vi "ReadTangoTestLongAttributes.vi"() -> ()   [LabVIEW 2009]
uses:
  tango_lv8/tango_vi.llb/ReadLongScalarAttribute.vi
  tango_lv8/tango_vi.llb/ReadLongSpectrumAttribute.vi
  tango_lv8/tango_vi.llb/ReadLongImageAttribute.vi
panel:
  out "?":bool
  out "scalar attr. read (RO)":i32
  out "Read/s":dbl
  in  "?":bool=TRUE
  out "Read/s":dbl
  out "Read/s":dbl
  in  "?":bool=TRUE
  in  "?":bool=TRUE
  out "Read/s":dbl
  in  "?":bool=TRUE
  out "error stack":string[](array[string])
  out "error stack":string[](array[string])
  out "error stack":string[](array[string])
  out "scalar attr. value":i32(graph)
  out "scalar attr. write value":i32
  out "scalar attr. read value":i32
  out "?":bool
  in  "attr_name":string="long_scalar"
  out "?":bool
  in  "attr_name":string="long_spectrum_ro"
  out "?":bool
  out "image attr. value":i32[][](graph)
  out "spectrum attr. value":i32[](graph)
  in  "attr_name":string="long_image_ro"
  in  "dev_name":string="tango/tangotest/1"
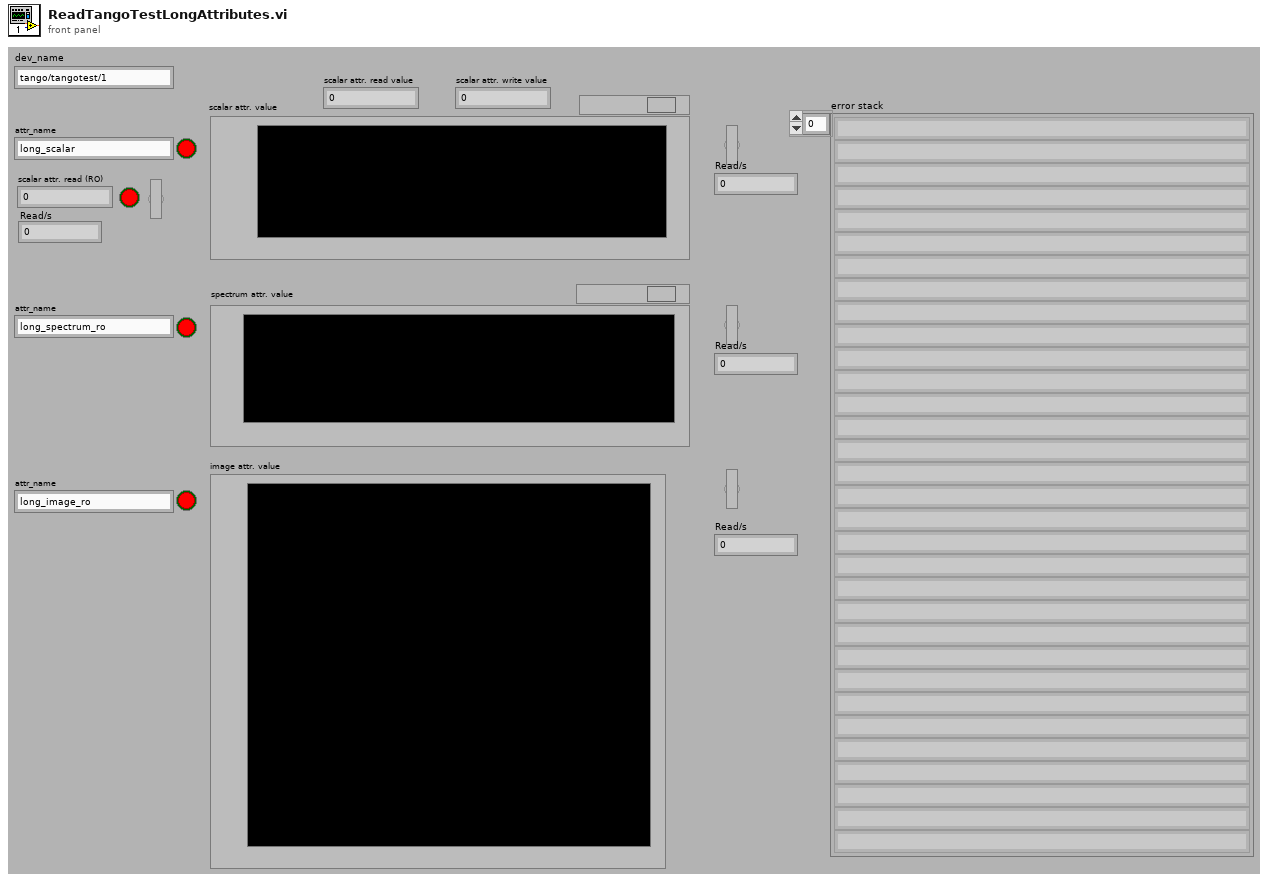
[diagram p1: front panel]
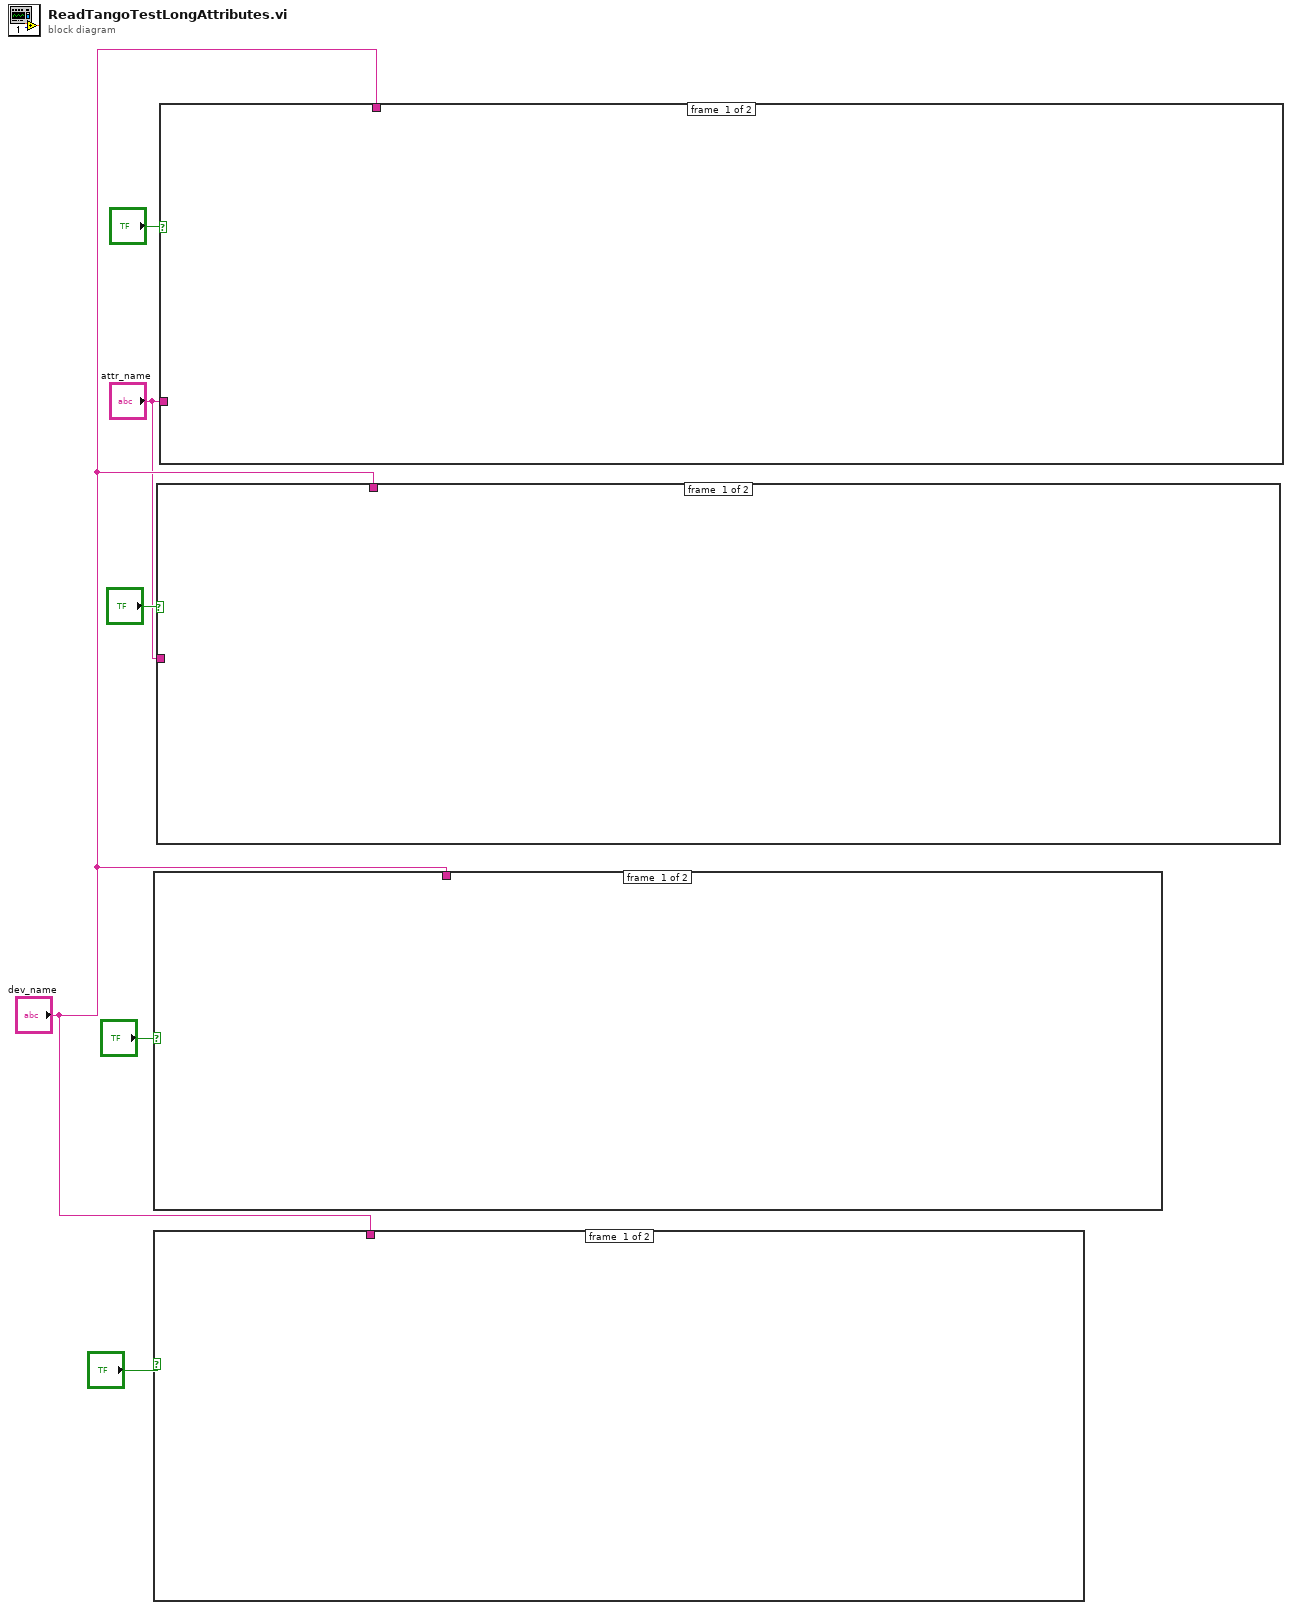
[diagram p0: block diagram]
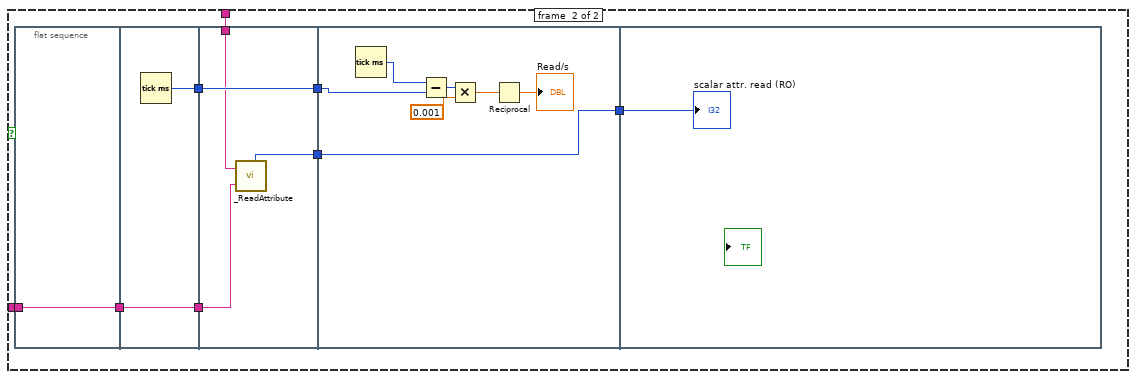
[diagram p2: hidden frame]
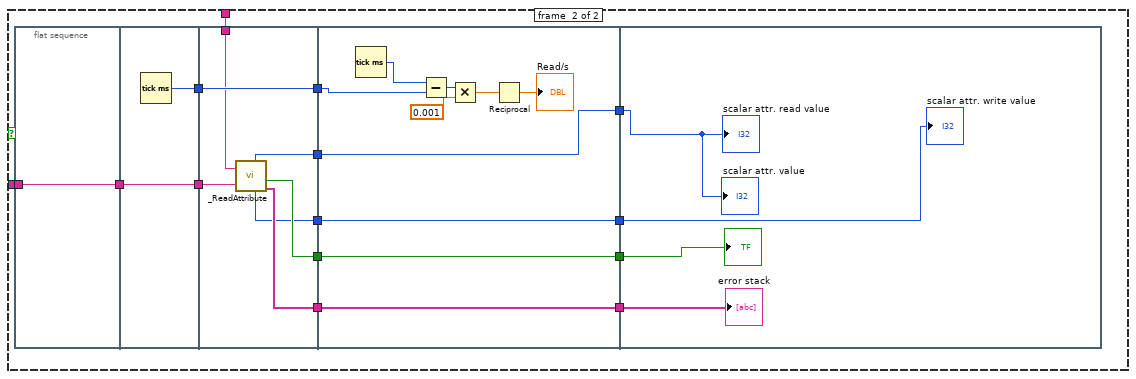
[diagram p3: hidden frame]
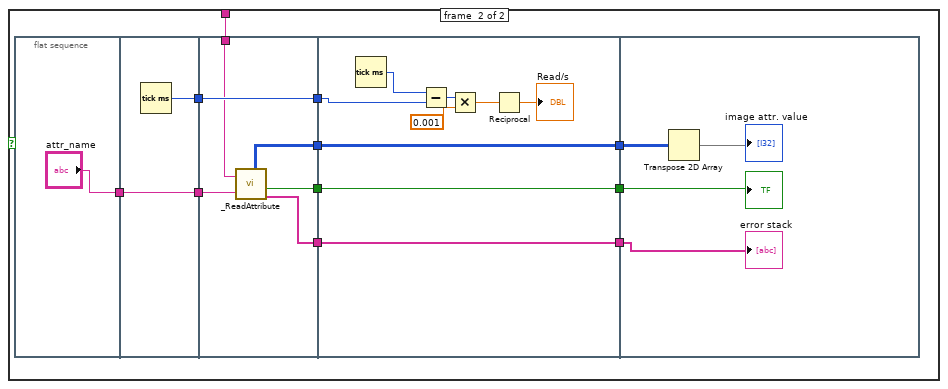
[diagram p4: hidden frame]
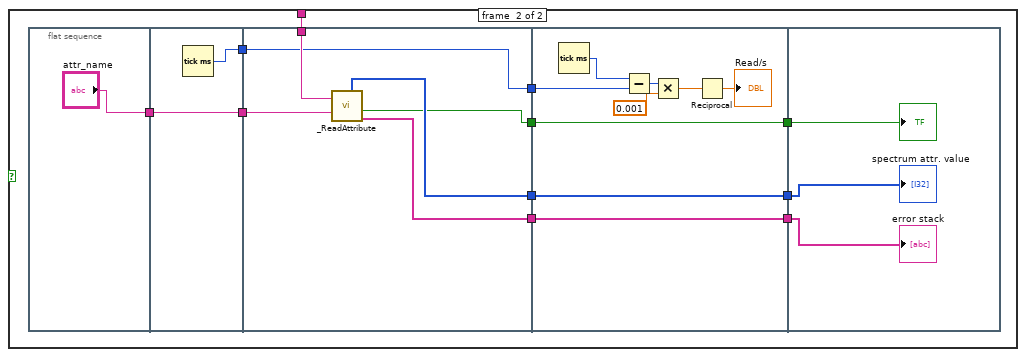
[diagram p5: hidden frame]
diagram:
  n1 = case shown="True" "?" {
    tunnel: "dev_name" -> [_ w9]
    frame #0 {
    }
    frame #1 {
      n2 = flat-sequence {
        tunnel: ["attr_name"] -> w17
        tunnel: [w20] -> w16
        tunnel: w17 -> [w20]
        tunnel: [w19] -> w15
        tunnel: w16 -> [w26]
        tunnel: w9 -> [w25]
        tunnel: w15 -> [w23]
        tunnel: [w22] -> w14
        tunnel: [w24] -> w13
        tunnel: [w23] -> w12
        tunnel: [w21] -> w7
        tunnel: [w33] -> w11
        tunnel: w14 -> [w33]
        tunnel: [w32] -> w10
        tunnel: w13 -> [w32]
        tunnel: w12 -> [w29]
        tunnel: [w27] -> w8
        tunnel: w7 -> [w27]
        tunnel: w11 -> [w37]
        tunnel: w10 -> [w38]
        tunnel: w8 -> [w36]
        frame #0 {
        }
        frame #1 {
          n3 = Tick Count (ms)() -> (millisecond timer value=w19:u32)
        }
        frame #2 {
          n4 = call-poly "_ReadAttribute.vi"("device name"=w25, "attribute name"=w26) -> ("value"=w22:i32[], "success"=w21:bool, "error stack"=w24:string[])  [unwired: 3 out]
        }
        frame #3 {
          n5 = Tick Count (ms)() -> (millisecond timer value=w30:u32)
          n6 = Subtract(x=w30, y=w29) -> (x-y=w35:u32)
          n7 = Multiply(x=w35, y=0.001) -> (x*y=w31:dbl)
          n8 = Reciprocal(x=w31) -> (1/x=→"Read/s":dbl)
        }
        frame #4 {
          "?" <- w36
          "spectrum attr. value" <- w37
          "error stack" <- w38
        }
      }
    }
  }
  n9 = case shown="True" "?" {
    tunnel: "dev_name" -> [_ w43]
    frame #0 {
    }
    frame #1 {
      n10 = flat-sequence {
        tunnel: ["attr_name"] -> w48
        tunnel: [w52] -> w49
        tunnel: w48 -> [w52]
        tunnel: [w51] -> w47
        tunnel: w49 -> [w58]
        tunnel: w47 -> [w57]
        tunnel: [w57] -> w46
        tunnel: [w56] -> w44
        tunnel: w43 -> [w55]
        tunnel: [w54] -> w41
        tunnel: [w53] -> w39
        tunnel: w46 -> [w62]
        tunnel: [w61] -> w45
        tunnel: w44 -> [w61]
        tunnel: [w60] -> w42
        tunnel: w41 -> [w60]
        tunnel: [w59] -> w40
        tunnel: w39 -> [w59]
        tunnel: w45 -> [w70]
        tunnel: w42 -> [w69]
        tunnel: w40 -> [w68]
        frame #0 {
        }
        frame #1 {
          n11 = Tick Count (ms)() -> (millisecond timer value=w51:u32)
        }
        frame #2 {
          n12 = call-poly "_ReadAttribute.vi"("device name"=w55, "attribute name"=w58) -> ("value"=w54:i32[][], "success"=w53:bool, "error stack"=w56:string[])  [unwired: 3 out]
        }
        frame #3 {
          n13 = Tick Count (ms)() -> (millisecond timer value=w63:u32)
          n14 = Subtract(x=w63, y=w62) -> (x-y=w67:u32)
          n15 = Multiply(x=w67, y=0.001) -> (x*y=w64:dbl)
          n16 = Reciprocal(x=w64) -> (1/x=→"Read/s":dbl)
        }
        frame #4 {
          n17 = Transpose 2D Array(2D array=w69) -> (transposed array=→"image attr. value":i32[][])
          "?" <- w68
          "error stack" <- w70
        }
      }
    }
  }
  n18 = case shown="True" "?" {
    tunnel: "dev_name" -> [_ w83]
    tunnel: "attr_name" -> [_ w74]
    frame #0 {
    }
    frame #1 {
      n19 = flat-sequence {
        tunnel: [w86] -> w75
        tunnel: w74 -> [w86]
        tunnel: [w88] -> w85
        tunnel: [w87] -> w76
        tunnel: w75 -> [w87]
        tunnel: w85 -> [w95]
        tunnel: [w95] -> w84
        tunnel: w83 -> [w92]
        tunnel: [w94] -> w81
        tunnel: [w93] -> w79
        tunnel: [w90] -> w77
        tunnel: w76 -> [w91]
        tunnel: [w89] -> w72
        tunnel: w84 -> [w100]
        tunnel: [w99] -> w82
        tunnel: w81 -> [w99]
        tunnel: [w98] -> w80
        tunnel: w79 -> [w98]
        tunnel: [w97] -> w78
        tunnel: w77 -> [w97]
        tunnel: [w96] -> w73
        tunnel: w72 -> [w96]
        tunnel: w82 -> [w106]
        tunnel: w80 -> [w109]
        tunnel: w78 -> [w108]
        tunnel: w73 -> [w107]
        frame #0 {
        }
        frame #1 {
          n20 = Tick Count (ms)() -> (millisecond timer value=w88:u32)
        }
        frame #2 {
          n21 = call-poly "_ReadAttribute.vi"("device name"=w92, "attribute name"=w91) -> ("value"=w94:i32, "setpoint"=w89:i32, "success"=w93:bool, "error stack"=w90:string[])  [unwired: 2 out]
        }
        frame #3 {
          n22 = Tick Count (ms)() -> (millisecond timer value=w101:u32)
          n23 = Subtract(x=w101, y=w100) -> (x-y=w105:u32)
          n24 = Multiply(x=w105, y=0.001) -> (x*y=w102:dbl)
          n25 = Reciprocal(x=w102) -> (1/x=→"Read/s":dbl)
        }
        frame #4 {
          "?" <- w109
          "scalar attr. read value" <- w106
          "scalar attr. value" <- w106
          "scalar attr. write value" <- w107
          "error stack" <- w108
        }
      }
    }
  }
  n26 = case shown="True" "?" {
    tunnel: "dev_name" -> [_ w115]
    tunnel: "attr_name" -> [_ w110]
    frame #0 {
    }
    frame #1 {
      n27 = flat-sequence {
        tunnel: [w118] -> w111
        tunnel: w110 -> [w118]
        tunnel: [w120] -> w117
        tunnel: [w119] -> w112
        tunnel: w111 -> [w119]
        tunnel: w117 -> [w124]
        tunnel: [w124] -> w116
        tunnel: w115 -> [w122]
        tunnel: [w123] -> w113
        tunnel: w112 -> [w121]
        tunnel: w116 -> [w126]
        tunnel: [w125] -> w114
        tunnel: w113 -> [w125]
        tunnel: w114 -> [w132]
        frame #0 {
        }
        frame #1 {
          n28 = Tick Count (ms)() -> (millisecond timer value=w120:u32)
        }
        frame #2 {
          n29 = call-poly "_ReadAttribute.vi"("device name"=w122, "attribute name"=w121) -> ("value"=w123:i32)  [unwired: 5 out]
        }
        frame #3 {
          n30 = Tick Count (ms)() -> (millisecond timer value=w127:u32)
          n31 = Subtract(x=w127, y=w126) -> (x-y=w131:u32)
          n32 = Multiply(x=w131, y=0.001) -> (x*y=w128:dbl)
          n33 = Reciprocal(x=w128) -> (1/x=→"Read/s":dbl)
        }
        frame #4 {
          "scalar attr. read (RO)" <- w132
        }
      }
    }
  }
